vi "Wire Multiple Objects Together.vi"(6 "Variant in":variant caption="变体输入", 7 "Shift Pressed?":bool caption="按下Shift？", 8 "error in (no error)":errorcluster caption="错误输入（无错误）", 10 "QD Combo Box Ref":refnum<vi> caption="快速放置组合框引用", 11 "QD Launch VI Ref":refnum<vi> caption="快速放置启动VI引用") -> (0 "error out":errorcluster caption="错误输出", 4 "Variant out":variant caption="变体输出")   [LabVIEW 2016]
doc: "连接程序框图上多个选中对象的匹配接线端。该快捷方式将从左至右连接对象匹配的数据类型。若同时按下[Shift]键，LabVIEW 将在连接选中对象后自动整理程序框图。\n\n默认快捷键-[W]"
uses:
  <vilib>/Utility/traverseref.llb/TRef TravTarget.ctl
  <resource>/dialog/QuickDrop/plugins/_WireMultipleSupport/What to Wire.ctl
  <vilib>/Utility/traverseref.llb/VI Scripting - Traverse.lvlib
panel:
  in  "Undo Name":string="连线多个对象" caption="撤消名称"
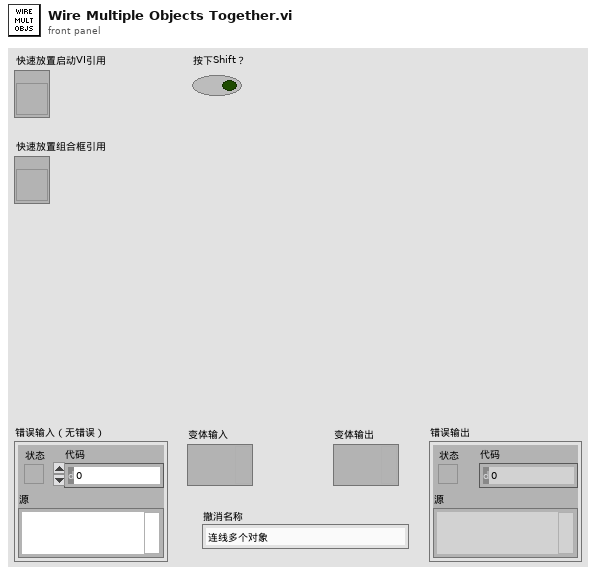
[diagram p1: front panel]
types:
  T1 = typedef "TRef TravTarget.ctl" = enum16{"FP", "BD", "Other"}
  T2 = typedef "What to Wire.ctl" = enum16{"node sinks", "node sources"}
  T3 = typedef "Node Terminal Info.ctl" = cluster{"Node Position (Left)":i32, "Node Ref":refnum<vi>, "Top Left":refnum<vi>, "Top Right":refnum<vi>, "Error Left":refnum<vi>, "Error Right":refnum<vi>}
  T4 = typedef "Available Non-Node.ctl" = cluster{"Left":i32, "Terminal":refnum<vi>}
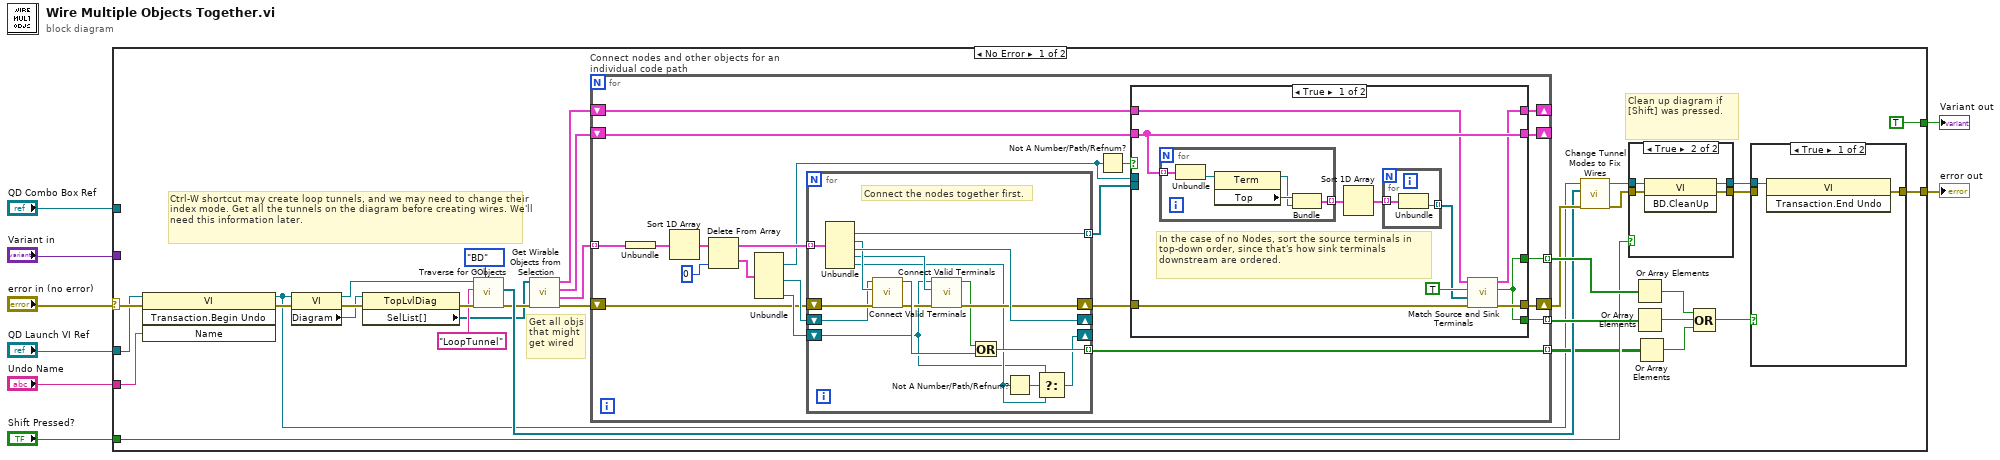
[diagram p0: block diagram]
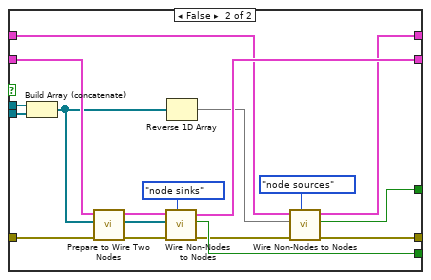
[diagram p2: hidden frame]
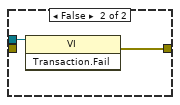
[diagram p4: hidden frame]
diagram:
  n1 = case shown="No Error" "error in (no error)" {
    selector: "error in (no error)" -> [w41 w124]
    tunnel: [w36 w124] -> w7
    tunnel: "QD Launch VI Ref" -> [w40 _]
    tunnel: "Shift Pressed?" -> [w27 _]
    tunnel: "QD Combo Box Ref" -> [_ _]
    tunnel: "Variant in" -> [_ _]
    tunnel: "Undo Name" -> [w39 _]
    tunnel: [TRUE _] -> w1
    frame No Error {
      # "Get all objs\nthat might\nget wired"
      # "Ctrl-W shortcut may create loop tunnels, and we may need to change their index mode. Get all the tunnels on the diagram before creating wires. We'll need this information later."
      # "Clean up diagram if [Shift] was pressed."
      n2 = invoke class="VI" method="Transaction.Begin Undo"(reference=w40, error in=w41, "Name"=w39) -> (reference out=w11:refnum<vi>, error out=w37:errorcluster)  [unwired: 1 in, 2 out]
      n3 = property class="VI"(reference=w11, error in=w37) -> (reference out=w21:refnum<vi>, error out=w35:errorcluster, "Diagram"=w34:refnum<vi>)
      n4 = property class="TopLvlDiag"(reference=w34, error in=w35) -> (error out=w33:errorcluster, "SelList[]"=w14:refnum<vi>[])  [unwired: 1 out]
      n5 = call <vilib>:"Traverse for GObjects.vi"("Traverse Target"=TRef_TravTarget."BD", "error in (no error)"=w33, "Class Name"="LoopTunnel", "VI Refnum"=w21) -> ("error out"=w18:errorcluster, "References"=w19:refnum<vi>[])  [unwired: 4 in, 2 out]
      n6 = call <resource>:"Get Wirable Objects from Selection.vi"("error in (no error)"=w18, "SelList[]"=w14) -> ("error out"=w13:errorcluster, "Parsed Selection List (Geographic Rows)"=w12:cluster{"Selection List":T3[]}[], "Controls, Constants, and Source Tunnels"=w15:T4[], "Indicators and Sink Tunnels"=w16:T4[])  [unwired: 6 in]
      n7 = for "Connect nodes and other objects for an individual code path" {
        tunnel: [w62] -> w31 mode=indexing
        tunnel: [w61] -> w28 mode=indexing
        tunnel: [w57] -> w17 mode=indexing
        shift-right: [w60] -> w25
        shift-left: w13 -> [w47]
        shift-right: [w46] -> _
        shift-left: w16 -> [w53]
        shift-right: [w45] -> _
        shift-left: w15 -> [w49]
        tunnel: w12 -> [w44] mode=indexing
        n8 = Unbundle(w44) -> ("Selection List"=w43:T3[])
        n9 = Sort 1D Array(array=w43) -> (sorted array=w56:T3[])
        n10 = Delete From Array(array=w56, index=0) -> (deleted portion=w59:T3, array with subset deleted=w58:T3[])  [unwired: 1 in]
        n11 = Unbundle(w59) -> ("Node Ref"=w50:refnum<vi>, "Top Right"=w52:refnum<vi>, "Error Right"=w51:refnum<vi>)  [unwired: 3 out]
        n12 = for {
          shift-right: [w105] -> w55
          shift-left: w47 -> [w109]
          tunnel: w58 -> [w113] mode=indexing
          shift-right: [w110] -> _
          shift-left: w52 -> [w102]
          tunnel: [w111] -> w57 mode=indexing
          tunnel: [w112] -> w54 mode=indexing
          shift-right: [w98] -> _
          shift-left: w51 -> [w99]
          # "Connect the nodes together first."
          n13 = Unbundle(w113) -> ("Node Ref"=w112:refnum<vi>, "Top Left"=w107:refnum<vi>, "Top Right"=w110:refnum<vi>, "Error Left"=w104:refnum<vi>, "Error Right"=w100:refnum<vi>)  [unwired: 1 out]
          n14 = call <resource>:"Connect Valid Terminals.vi"("error in (no error)"=w109, "Sink Term"=w107, "Source Term"=w102) -> ("error out"=w106:errorcluster, "Connection Made?"=w108:bool)  [unwired: 7 in]
          n15 = call <resource>:"Connect Valid Terminals.vi"("error in (no error)"=w106, "Sink Term"=w104, "Source Term"=w99) -> ("error out"=w105:errorcluster, "Connection Made?"=w103:bool)  [unwired: 7 in]
          n16 = Or(x=w103, y=w108) -> (x .or. y?=w111:bool)
          n17 = Not A Number/Path/Refnum?(number/path/refnum=w100) -> (NaN/Path/Refnum?=w101:bool)
          n18 = Select(t=w99, s=w101, f=w100) -> (s? t:f=w98:refnum<vi>)
        }
        n19 = Not A Number/Path/Refnum?(number/path/refnum=w50) -> (NaN/Path/Refnum?=w48:bool)
        n20 = case shown="True" w48 {
          tunnel: w55 -> [w71 w86]
          tunnel: w54 -> [_ w84]
          tunnel: [w66 w95] -> w62
          tunnel: [w66 w87] -> w61
          tunnel: w53 -> [w69 w89]
          tunnel: [w70 w92] -> w60
          tunnel: w50 -> [_ w97]
          tunnel: w49 -> [w72 w83]
          tunnel: [w68 w88] -> w46
          tunnel: [w72 w96] -> w45
          frame True {
            # "In the case of no Nodes, sort the source terminals in top-down order, since that's how sink terminals downstream are ordered."
            n21 = for {
              tunnel: w72 -> [w79] mode=indexing
              tunnel: [w75] -> w65 mode=indexing
              n22 = Unbundle(w79) -> ("Terminal"=w78:refnum<vi>)  [unwired: 1 out]
              n23 = property class="Term"(reference=w78) -> (reference out=w76:refnum<vi>, "Top"=w77:i32)  [unwired: 1 in, 1 out]
              n24 = Bundle("Top"=w77, "Terminal"=w76) -> (w75:cluster{"Top":i32, "Terminal":refnum<vi>})  [unwired: 1 in]
            }
            n25 = Sort 1D Array(array=w65) -> (sorted array=w64:cluster{"Top":i32, "Terminal":refnum<vi>}[])
            n26 = for {
              tunnel: w64 -> [w74] mode=indexing
              tunnel: [w73] -> w63 mode=indexing
              n27 = Unbundle(w74) -> ("Terminal"=w73:refnum<vi>)  [unwired: 1 out]
            }
            n28 = call <resource>:"Match Source and Sink Terminals.vi"("error in (no error)"=w71, "Node Terminals"=w63, "Node Sources?"=TRUE, "Available Non-Nodes in"=w69) -> ("error out"=w70:errorcluster, "Any Changes?"=w66:bool, "Available Non-Nodes out"=w68:T4[])  [unwired: 5 in]
          }
          frame False {
            n29 = Build Array (concatenate)(w97, w84) -> (w81:refnum<vi>[])
            n30 = call <resource>:"Prepare to Wire Two Nodes.vi"("error in (no error)"=w86, "Nodes"=w81, "Available Non-Nodes in"=w83) -> ("error out"=w85:errorcluster, "dup Nodes"=w80:refnum<vi>[], "Available Non-Nodes out"=w82:T4[])  [unwired: 6 in]
            n31 = call <resource>:"Wire Non-Nodes to Nodes.vi"("What to Wire"=What_to_Wire."node sinks", "error in (no error)"=w85, "Nodes"=w80, "Available Non-Nodes in"=w82) -> ("error out"=w93:errorcluster, "Any Changes?"=w95:bool, "Available Non-Nodes out"=w96:T4[])  [unwired: 5 in]
            n32 = Reverse 1D Array(array=w81) -> (reversed array=w90:refnum<vi>[])
            n33 = call <resource>:"Wire Non-Nodes to Nodes.vi"("What to Wire"=What_to_Wire."node sources", "error in (no error)"=w93, "Nodes"=w90, "Available Non-Nodes in"=w89) -> ("error out"=w92:errorcluster, "Any Changes?"=w87:bool, "Available Non-Nodes out"=w88:T4[])  [unwired: 5 in]
          }
        }
      }
      n34 = call <resource>:"Change Tunnel Modes to Fix Wires.vi"("error in (no error)"=w25, "All Tunnels (before wiring)"=w19, "VI"=w11) -> ("error out"=w24:errorcluster, "dup VI"=w10:refnum<vi>)  [unwired: 7 in]
      n35 = case shown="True" w27 {
        tunnel: w24 -> [w115 w119]
        tunnel: [w115 w118] -> w9
        tunnel: w10 -> [w114 w117]
        tunnel: [w114 w116] -> w26
        frame False {
        }
        frame True {
          n36 = invoke class="VI" method="BD.CleanUp"(reference=w117, error in=w119) -> (reference out=w116:refnum<vi>, error out=w118:errorcluster)  [unwired: 1 in, 1 out]
        }
      }
      n37 = Or Array Elements(Boolean array=w28) -> (logical OR=w29:bool)
      n38 = Or Array Elements(Boolean array=w31) -> (logical OR=w30:bool)
      n39 = Or Array Elements(Boolean array=w17) -> (logical OR=w20:bool)
      n40 = Compound Arithmetic op=OR(w29, w30, w20) -> (w32:bool)
      n41 = case shown="True" w32 {
        tunnel: w26 -> [w120 w122]
        tunnel: [w121 w123] -> w36
        tunnel: w9 -> [_ _]
        frame True {
          n42 = invoke class="VI" method="Transaction.End Undo"(reference=w120) -> (error out=w121:errorcluster)  [unwired: 2 in, 2 out]
        }
        frame False {
          n43 = invoke class="VI" method="Transaction.Fail"(reference=w122) -> (error out=w123:errorcluster)  [unwired: 2 in, 2 out]
        }
      }
    }
    frame Error {
    }
  }
  "error out" <- w7
  "Variant out" <- w1
